vi "Configure Schedule Text.vi"(0 "VISA resource name":refnum<visa-resource-name>, 1 "Schedule Number (1)":i32=1 min=1 max=12 step=1, 2 "Title (\"\")":string, 3 "Notification Message1 (\"\")":string, 4 "Notification Message2 (\"\")":string, 5 "error in (no error)":errorcluster) -> (14 "VISA resource name out":refnum<visa-resource-name>, 19 "error out":errorcluster)   [LabVIEW 2020, in "Yokogawa GX Series.lvlib"]
doc: "Sets the notification contents.\n\nCommand: SScheduleText"
uses:
  <instrlib>/Yokogawa GX Series/Yokogawa GX Series.lvlib
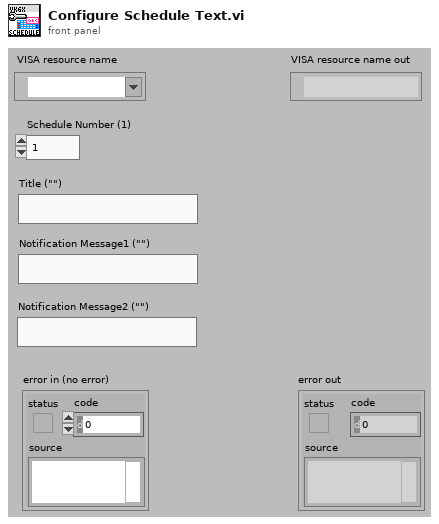
[diagram p1: front panel]
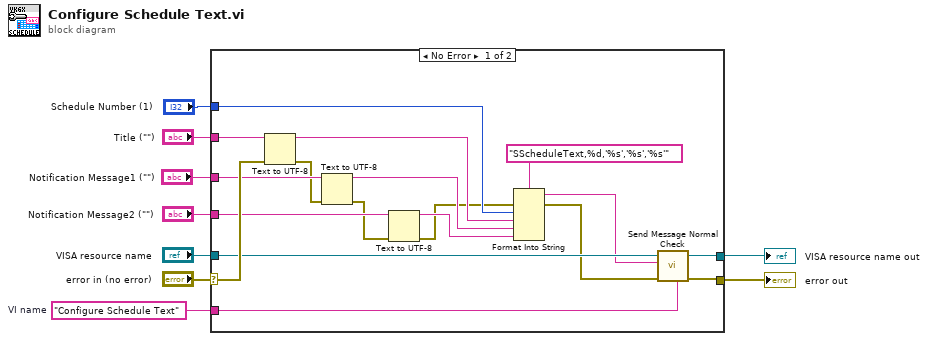
[diagram p0: block diagram]
diagram:
  w6 = "Configure Schedule Text"  # VI name
  n1 = case shown="No Error" "error in (no error)" {
    selector: "error in (no error)" -> [w21 w28]
    tunnel: "VISA resource name" -> [w12 w29]
    tunnel: [w27 w29] -> w8
    tunnel: [w26 w28] -> w7
    tunnel: w6 -> [w25 _]
    tunnel: "Schedule Number (1)" -> [w23 _]
    tunnel: "Title (\"\")" -> [w22 _]
    tunnel: "Notification Message1 (\"\")" -> [w20 _]
    tunnel: "Notification Message2 (\"\")" -> [w19 _]
    frame No Error {
      n2 = Text to UTF-8(8:w21, 11:w22) -> (0:w15:errorcluster, 3:w18:string)  [unwired: 1 in]
      n3 = Text to UTF-8(8:w15, 11:w20) -> (0:w14:errorcluster, 3:w17:string)  [unwired: 1 in]
      n4 = Text to UTF-8(8:w14, 11:w19) -> (0:w13:errorcluster, 3:w16:string)  [unwired: 1 in]
      n5 = Format Into String(format string="SScheduleText,%d,'%s','%s','%s'", error in=w13, w23, w18, w17, w16) -> (resulting string=w10:string, error out=w11:errorcluster)  [unwired: 1 in]
      n6 = call <instrlib>:"Send Message Normal Check.vi"("Source (\"\")"=w25, "error in (no error)"=w11, "Send Message (\"\")"=w10, "VISA resource name"=w12) -> ("error out"=w26:errorcluster, "VISA resource name out"=w27:refnum<visa-resource-name>)  [unwired: 2 in, 4 out]
    }
    frame Error {
    }
  }
  "error out" <- w7
  "VISA resource name out" <- w8
